vi "ROI entry-Obtain image arrays.vi"(8 "error in (no error)":errorcluster) -> (0 "error IO":errorcluster, 3 "RedImageArray":T1[](array[typedef]))   [LabVIEW 2020]
uses:
  <vilib>/vision/Image Controls.llb/IMAQ Image.ctl
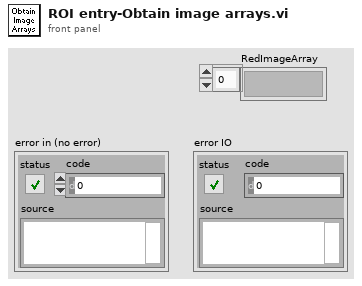
[diagram p1: front panel]
types:
  T1 = typedef "IMAQ Image.ctl" = refnum<image>
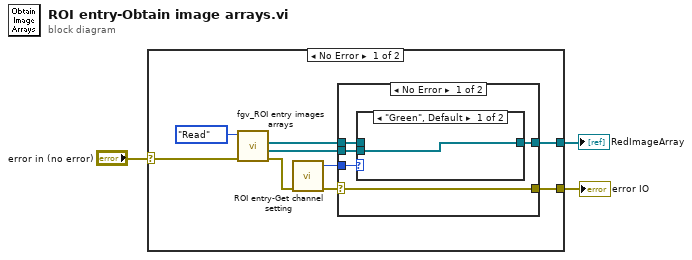
[diagram p0: block diagram]
diagram:
  n1 = case shown="No Error" "error in (no error)" {
    selector: "error in (no error)" -> [w5 w21]
    tunnel: [w7 _] -> w3
    tunnel: [w4 w21] -> w1
    frame No Error {
      n2 = call "fgv_ROI entry images arrays.vi"("error in (no error)"=w5, "Function"=enum16{"Intialize", "Write", "Read", "Clear"}."Read") -> ("error out"=w12:errorcluster, "GreenImageArray"=w11:T1[], "RedImageArray"=w10:T1[])  [unwired: 7 in]
      n3 = call "ROI entry-Get channel setting.vi"("error in (no error)"=w12) -> ("error out"=w6:errorcluster, "Selected channel"=w8:enum16{"Green", "Red"})  [unwired: 9 in]
      n4 = case shown="No Error" w6 {
        selector: w6 -> [w13 w20]
        tunnel: w11 -> [w17 _]
        tunnel: w10 -> [w16 _]
        tunnel: w8 -> [w15 _]
        tunnel: [w14 _] -> w7
        tunnel: [w13 w20] -> w4
        frame No Error {
          n5 = case shown="\"Green\", Default" w15 {
            tunnel: [w18 w19] -> w14
            tunnel: w16 -> [_ w19]
            tunnel: w17 -> [w18 _]
            frame "Green", Default {
            }
            frame "Red" {
            }
          }
        }
        frame Error {
        }
      }
    }
    frame Error {
    }
  }
  "RedImageArray" <- w3
  "error IO" <- w1
